vi "Loop Error Stop.vi"(8 "error in":errorcluster, 11 "user event":refnum<user-event>) -> (0 "error out":errorcluster)   [LabVIEW 2021]
doc: "This VI helps to stop the program if there is an error in the DAQ, File and Data Display Loop."
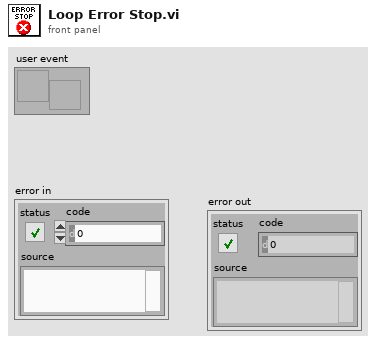
[diagram p1: front panel]
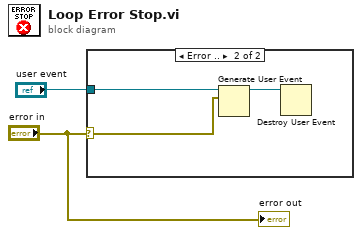
[diagram p0: block diagram]
diagram:
  n1 = case shown="Error .." "error in" {
    selector: "error in" -> [_ w3]
    tunnel: "user event" -> [_ w4]
    frame No Error {
    }
    frame Error {
      n2 = Generate User Event(user event=w4, event data cluster=w3) -> (user event out=w5:refnum<user-event>)  [unwired: 2 in, 1 out]
      n3 = Destroy User Event(user event=w5) -> ()  [unwired: 1 in, 1 out]
    }
  }
  "error out" <- "error in"
